vi "SW_Add_or_Modify_Reward_Condition_2.vi"(3 "Array of conditions out":T12, 6 "IO parameters cluster":T1, 7 "Add or Modify?":enum16{"Add", "Modify"}(ring), 8 "error in (no error)":T15, 9 "Main Tree Control in":refnum<vi>, 10 "Calibration parameters":T13={"Timing calibration sw/hw"=1.0, "True FPS"=80.0, "True frame time, s"=0.0125, "Disp. calibration info"=[]} {"True frame time, s" format="%.10g"; "Disp. calibration info"."Speed, µl per ms" format="%.3g"; "True FPS" format="%.10g"; "Timing calibration sw/hw" format="%.10g"}, 11 "Array of conditions in":T12) -> (0 "error out":T15, 1 "Main Tree Control out":refnum<vi>)   [LabVIEW 2018, in "Tracker.lvlib"]
uses:
  Tracker.lvlib
  <vilib>/Utility/miscctls.llb/LVPointTypeDef.ctl
  Controls/CTL_Dispenser_calibration_info.ctl
  Controls/CTL_Calibration_parameters.ctl
  Classes/Reward_Condition/Reward_Condition.lvclass
  Classes/Reward_Condition/Controls/RC_Array_of_Conditions.ctl
  Controls/CTL_Conditions_build_parameters_2.ctl
  Controls/CTL_Condition_type.ctl
  Controls/CTL_Comparison_type.ctl
  Controls/CTL_Validity_check_criteria.ctl
  Controls/CTL_Condition_response_type.ctl
  Controls/CTL_Conditions_Cluster.ctl
  Controls/CTL_IO_params_cluster.ctl
  Controls/CTL_Reponse_port_info.ctl
  Controls/CTL_Response_info.ctl
panel:
  out "Local tree ref":refnum<vi>
  in  "Discard and exit":bool
  in  "Reset Button":bool
  out "Index of selected condition":i32
  out "Has been set":bool
  in  "Specifiers On/Off":T2
  in  "Save and exit":bool
  out "Validity criteria(s)":T4(array[cluster])
  out "Subcondition":T5={"Enabled"=FALSE, "Name"="", "Specifier(s)"=[], "Response"={"Response type"=enum."Air puff", "TTL port"=enum."Port 1", "TTL pulse length, ms"=0.0}, "Has been set"=FALSE} caption="Condition" {"Specifier(s)"."Validity criteria(s)"."Validity value" min=0.0 step=0.1 format="%.2g"; "Specifier(s)"."Value" step=1.0 format="%#.2g"}
  in  "TTL pulse length":dbl caption="No output"
  in  "TTL port":T10
  in  "Response type":T9=enum."Air puff"
  in  "Valid for, units":dbl caption="Has been True for, units" format="%.2g"
  in  "Validity Enabled":bool caption="Enabled"
  in  "SC. Validity Criteria":T3 caption="Validity Criteria"
  in  "Compare against":dbl
  in  "Comparison type":T7
  in  "SubCondition type":T6
  in  "Subcondition #":i32(slide)=5 min=1 max=5 step=1 scale=5.0..1.0
  in  "Specifier(s)":T11(array[cluster])
  in  "C. Name":string caption="Condition Name"
  out "Cond. work index":i32
  in  "C. Enabled":bool caption="Enabled"
  out "Review changes before save":string(tree) caption="Reward and stimulation out"
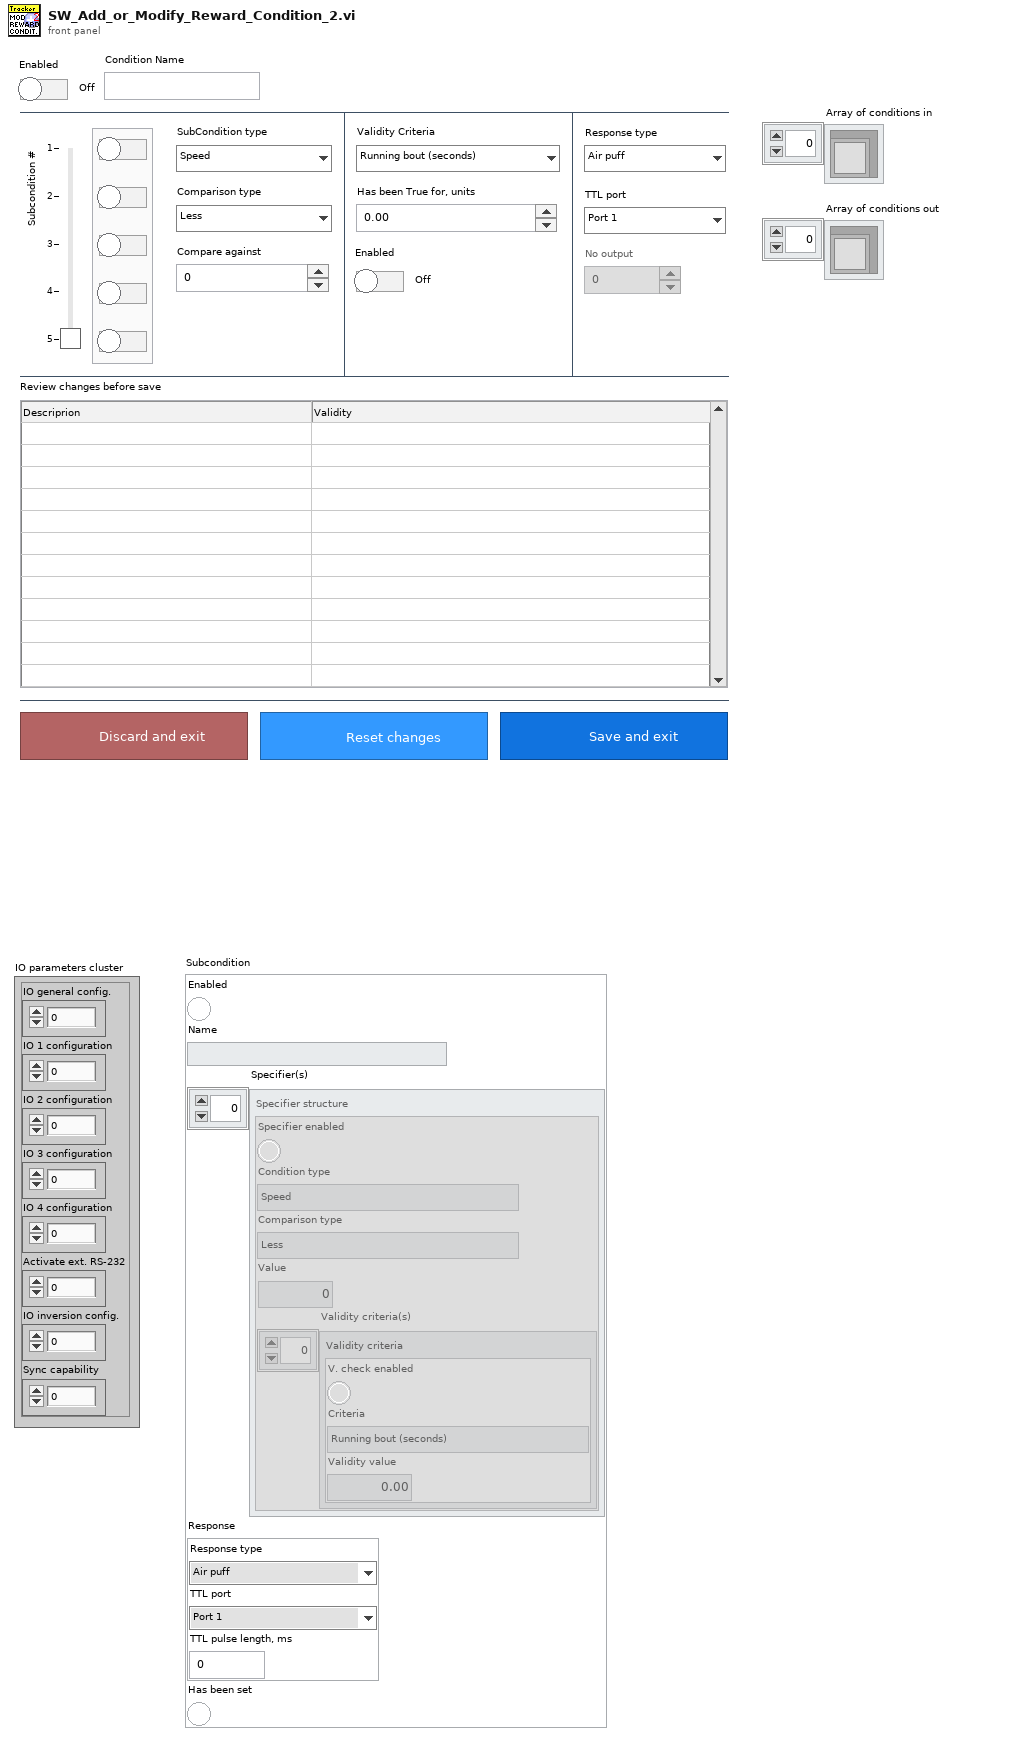
[diagram p1: front panel]
types:
  T1 = typedef "Tracker.lvlib/CTL_IO_params_cluster.ctl" = cluster{"IO general config.":u16, "IO 1 configuration":u16, "IO 2 configuration":u16, "IO 3 configuration":u16, "IO 4 configuration":u16, "Activate ext. RS-232":u16, "IO inversion config.":u16, "Sync capability":u8}
  T2 = cluster{"Specifier on/off":bool, "Specifier on/off 2":bool, "Specifier on/off 3":bool, "Specifier on/off 4":bool, "Specifier on/off 5":bool}
  T3 = typedef "Tracker.lvlib/CTL_Validity_check_criteria.ctl" = enum16{"Running bout (seconds)", "Running bout (meters)"}
  T4 = cluster{"V. check enabled":bool, "Criteria":T3, "Validity value":dbl}[]
  T5 = typedef "Tracker.lvlib/CTL_Conditions_Cluster.ctl" = cluster{"Enabled":bool, "Name":string, "Specifier(s)":cluster{"Specifier enabled":bool, "Condition type":T6, "Comparison type":T7, "Value":dbl, "Validity criteria(s)":cluster{"V. check enabled":bool, "Criteria":T3, "Validity value":dbl}[]}[], "Response":T8, "Has been set":bool}
  T6 = typedef "Tracker.lvlib/CTL_Condition_type.ctl" = enum16{"Speed", "Zone", "Angle to wall"}
  T7 = typedef "Tracker.lvlib/CTL_Comparison_type.ctl" = enum16{"Less", "Less or Equal", "Equal", "Greater or Equal", "Greater", "Not Equal"}
  T8 = typedef "Tracker.lvlib/CTL_Response_info.ctl" = cluster{"Response type":T9, "TTL port":T10, "TTL pulse length, ms":dbl}
  T9 = typedef "Tracker.lvlib/CTL_Condition_response_type.ctl" = enum16{"None", "Air puff", "Liquid reward"}
  T10 = typedef "Tracker.lvlib/CTL_Reponse_port_info.ctl" = enum16{"Port 1", "Port 2", "Port 3", "Port 4"}
  T11 = cluster{"Specifier enabled":bool, "Condition type":T6, "Comparison type":T7, "Value":dbl, "Validity criteria(s)":cluster{"V. check enabled":bool, "Criteria":T3, "Validity value":dbl}[]}[]
  T12 = typedef "Tracker.lvlib/Reward_Condition.lvclass/RC_Array_of_Conditions.ctl" = refnum<class "Reward_Condition.lvclass">[]
  T13 = typedef "Tracker.lvlib/CTL_Calibration_parameters.ctl" = cluster{"Timing calibration sw/hw":dbl, "True FPS":dbl, "True frame time, s":dbl, "Disp. calibration info":T14}
  T14 = typedef "Tracker.lvlib/CTL_Dispenser_calibration_info.ctl" = cluster{"Channel":u8, "Speed, µl per ms":dbl}[]
  T15 = cluster{"Boolean Round":bool, "code":i32, "source":string}
  T16 = typedef "LVPointTypeDef.ctl" = cluster{"Horizontal":i16, "Vertical":i16}
  T17 = typedef "Tracker.lvlib/CTL_Conditions_build_parameters_2.ctl" = cluster{"TreeControl":refnum<vi>, "TTL pulse length ref":refnum<vi>, "Array of conditions":T12, "Condition working index":i32, "Subcondition #":i32, "Calibration parameters":T13}
  T18 = cluster{"[0]":bool, "[1]":bool, "[2]":bool, "[3]":bool, "[4]":bool}
  T19 = cluster{"Specifier enabled":bool, "Condition type":T6, "Comparison type":T7, "Value":dbl, "Validity criteria(s)":cluster{"V. check enabled":bool, "Criteria":T3, "Validity value":dbl}[]}
  T20 = cluster{"V. check enabled":bool, "Criteria":T3, "Validity value":dbl}
  T21 = cluster{"Specifiers On/Off[0]":bool, "Specifiers On/Off[1]":bool, "Specifiers On/Off[2]":bool, "Specifiers On/Off[3]":bool, "Specifiers On/Off[4]":bool}
  T22 = cluster{"Validity Enabled":bool, "SC. Validity Criteria":T3, "Valid for, units":dbl}
  T23 = cluster{"Response type":T9, "TTL port":T10, "TTL pulse length, ms out":dbl}
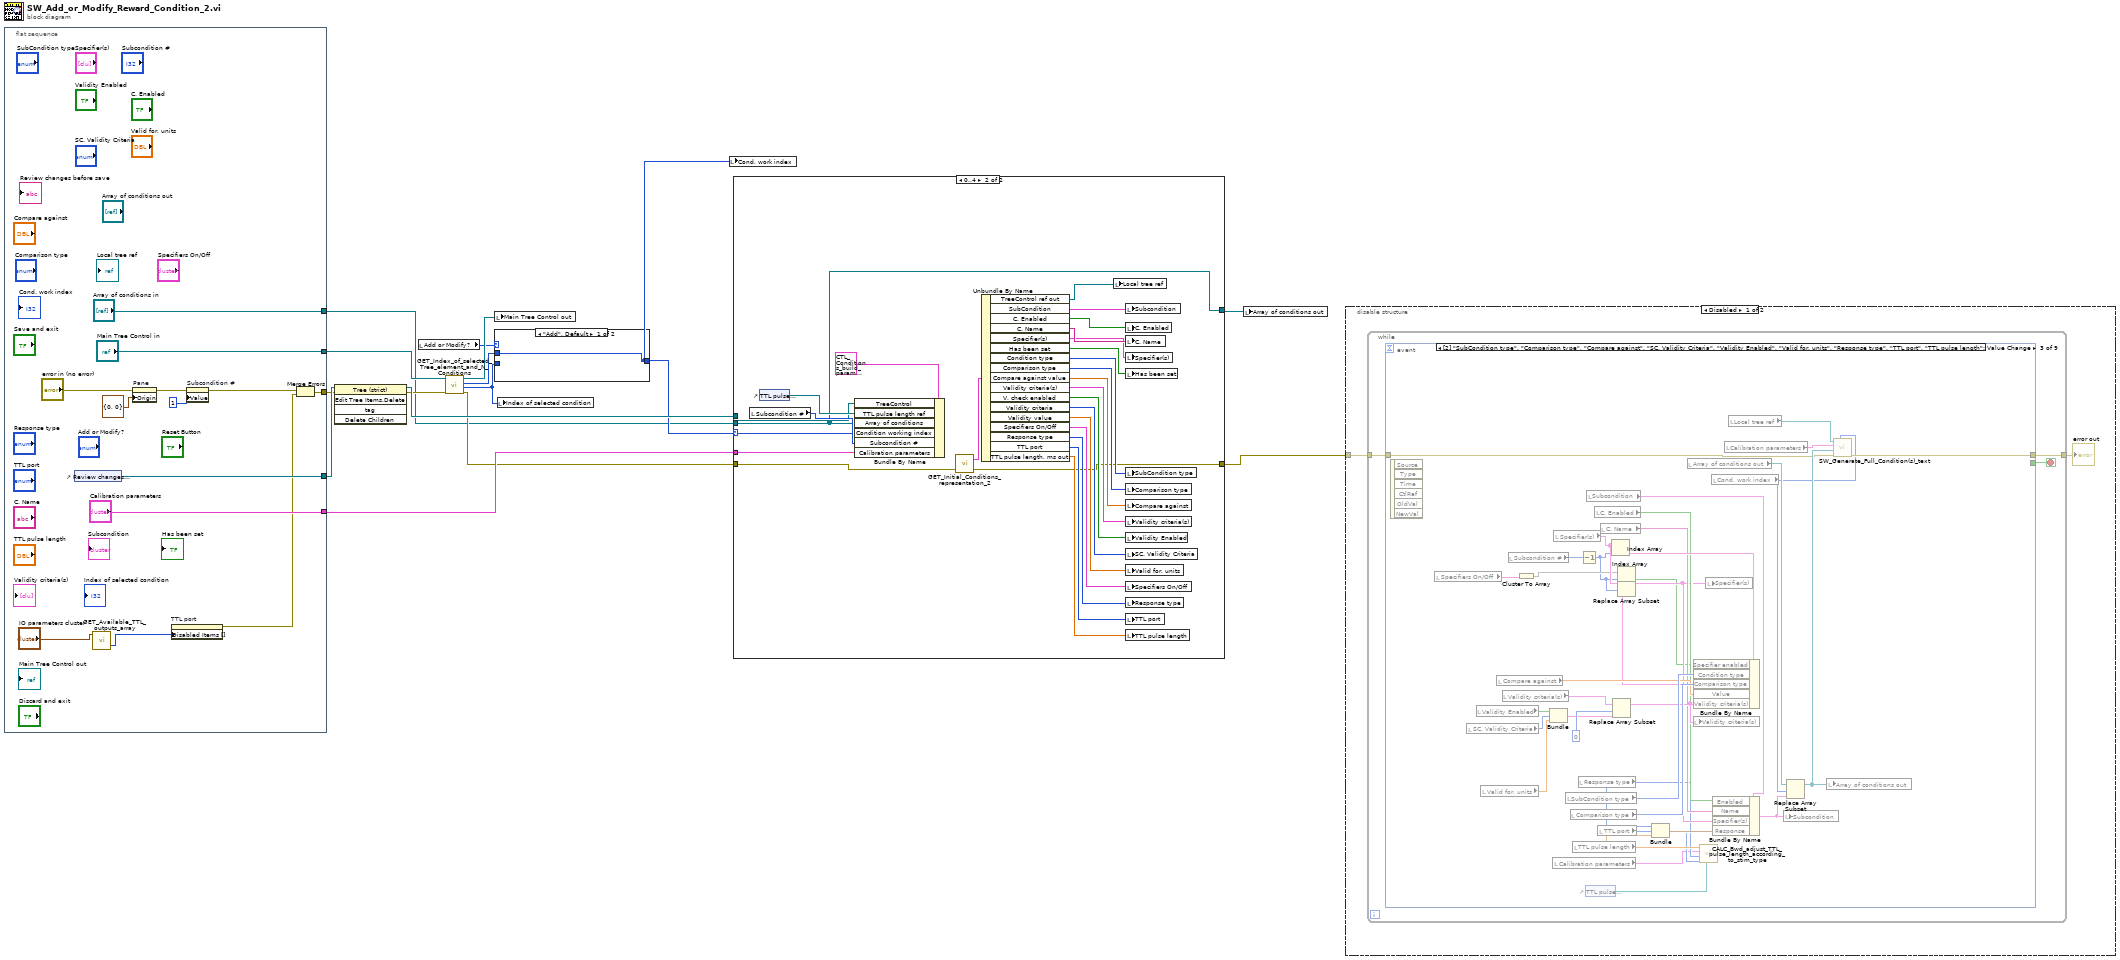
[diagram p0: block diagram]
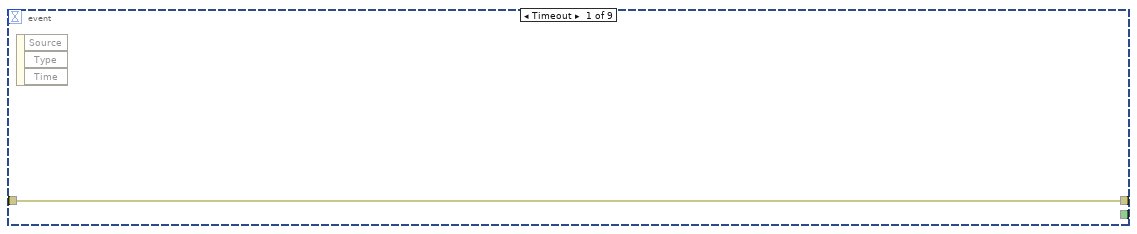
[diagram p2: hidden frame]
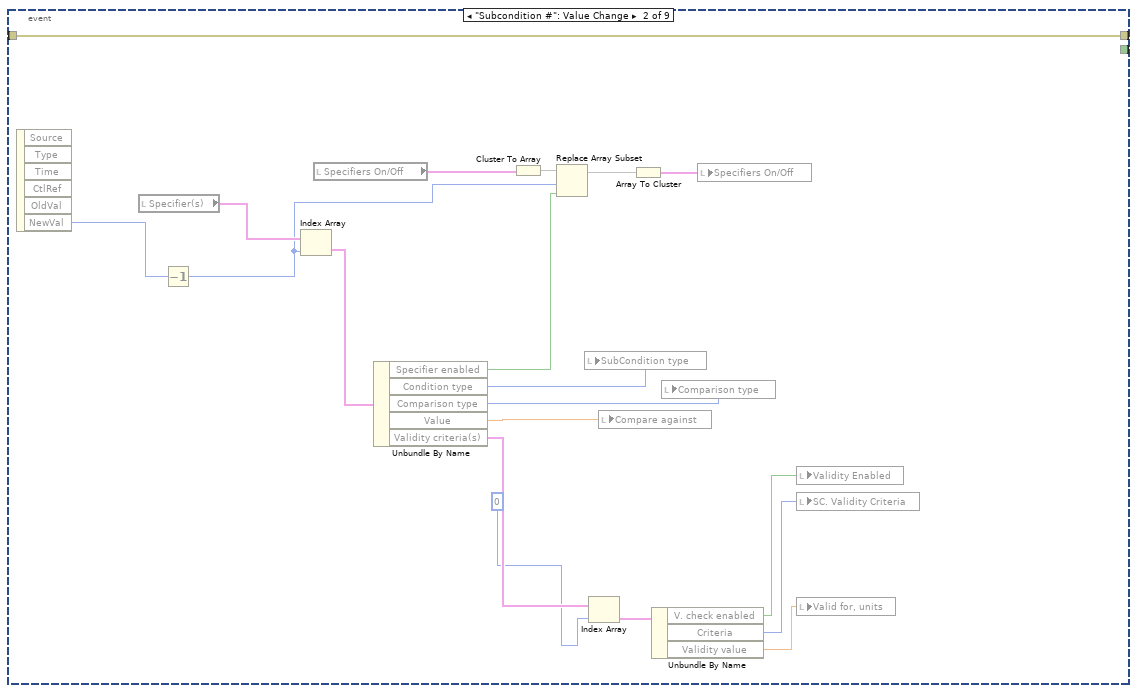
[diagram p3: hidden frame]
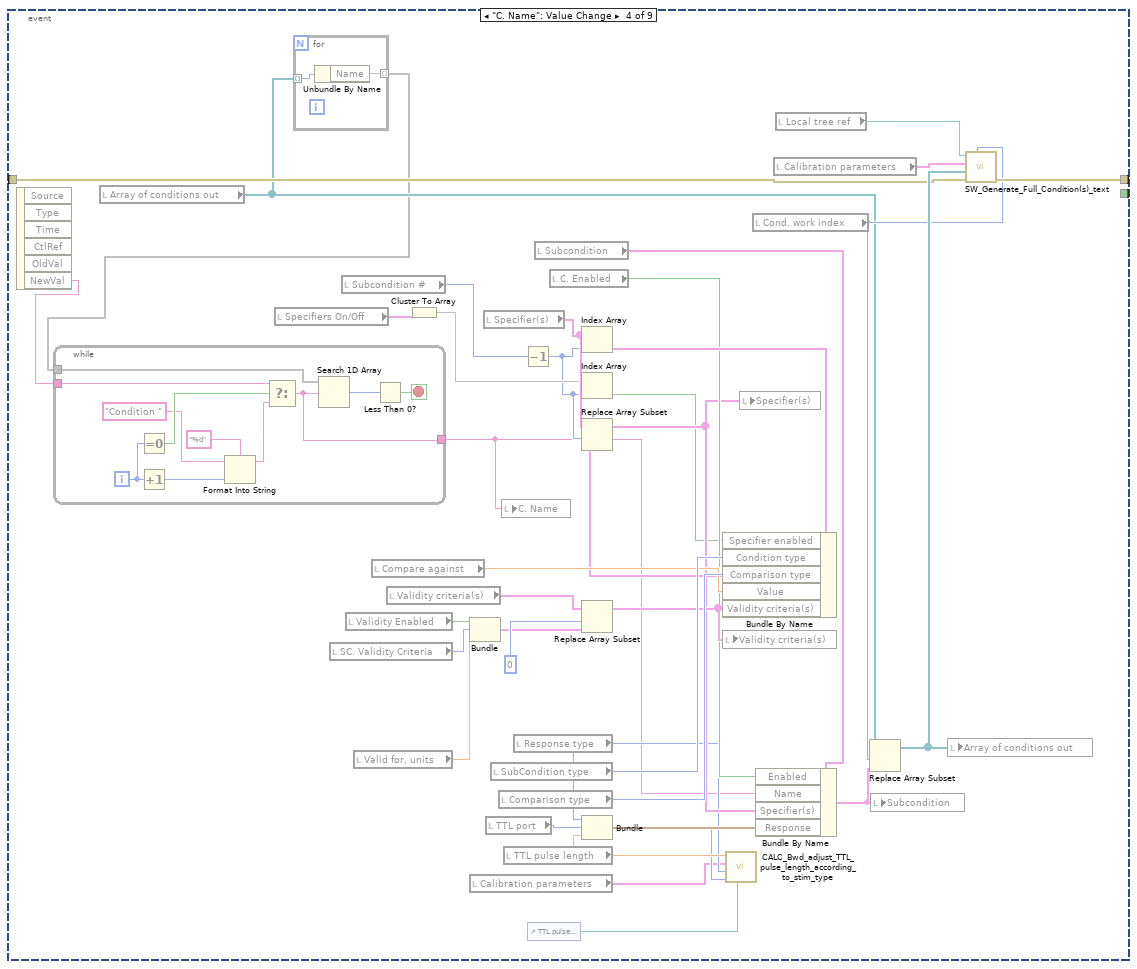
[diagram p4: hidden frame]
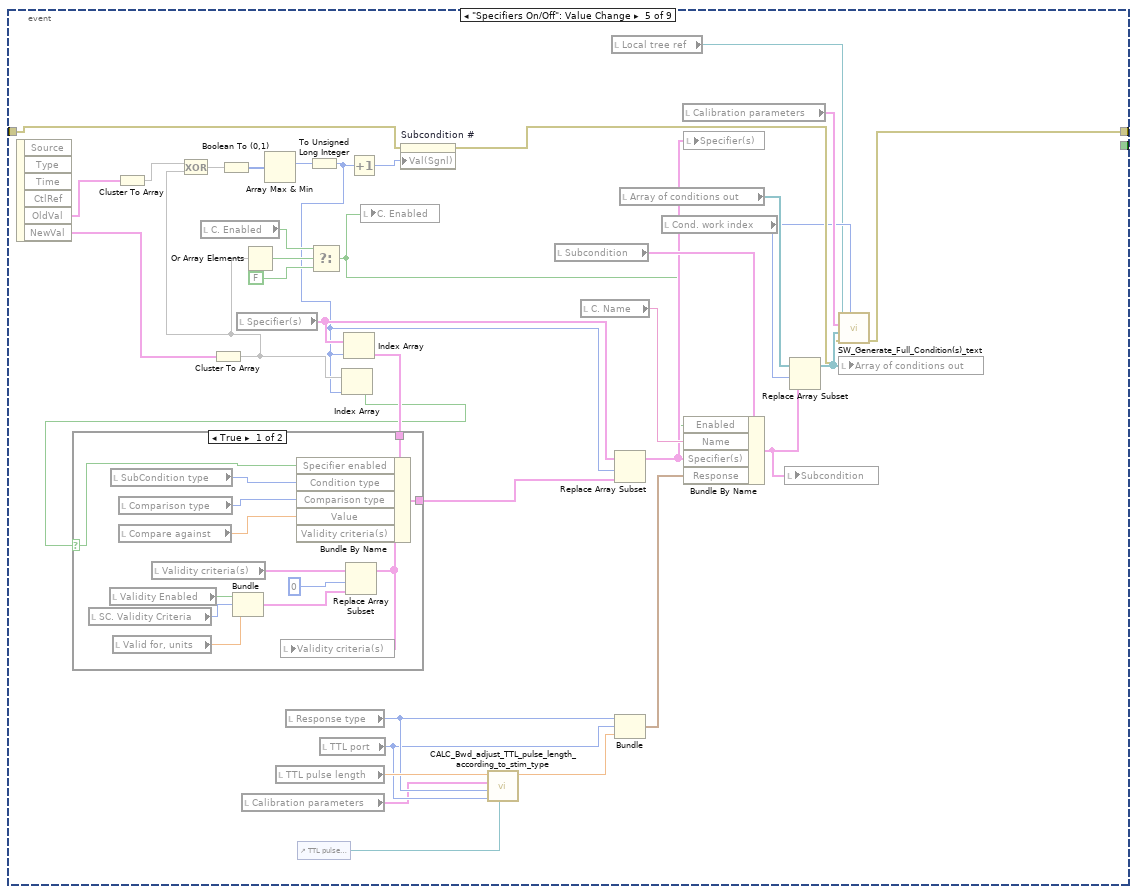
[diagram p5: hidden frame]
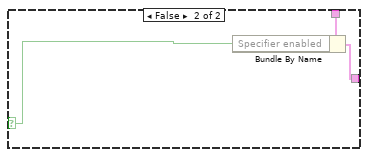
[diagram p6: hidden frame]
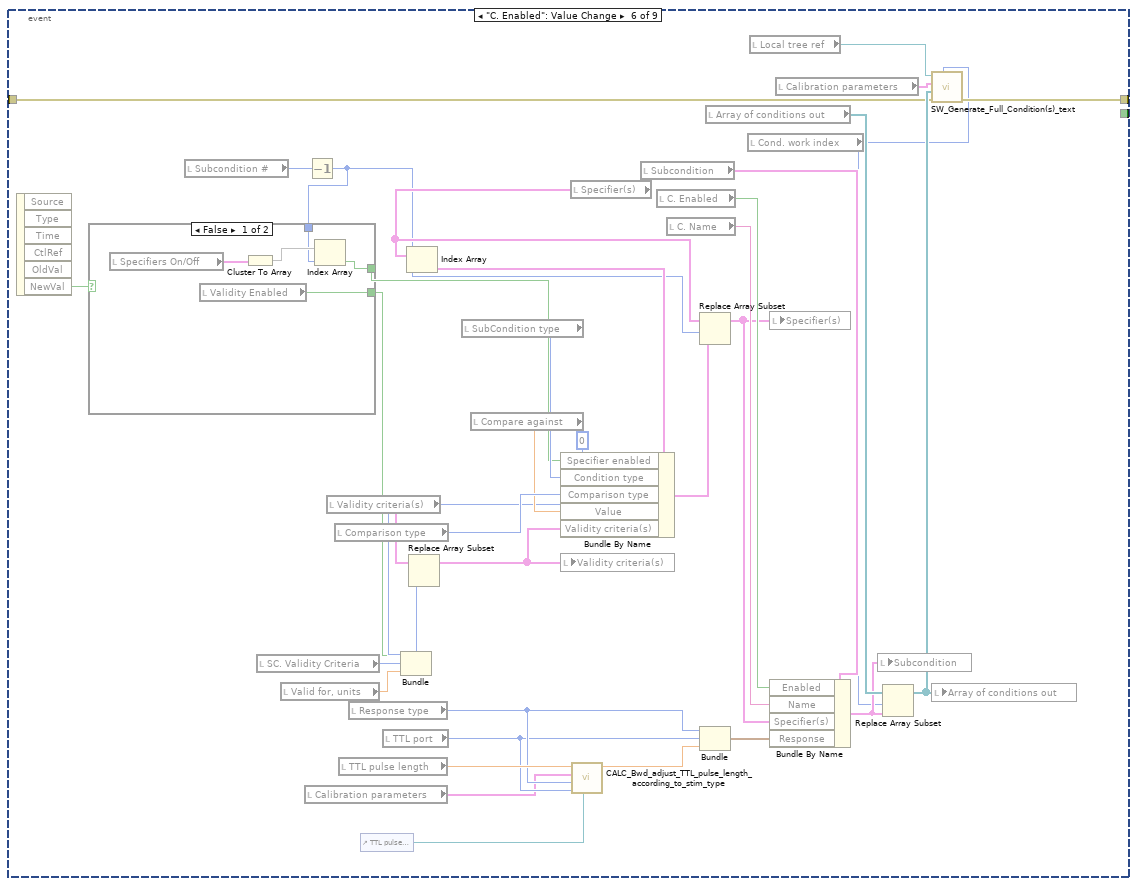
[diagram p7: hidden frame]
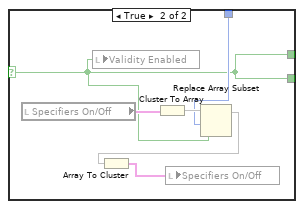
[diagram p8: hidden frame]
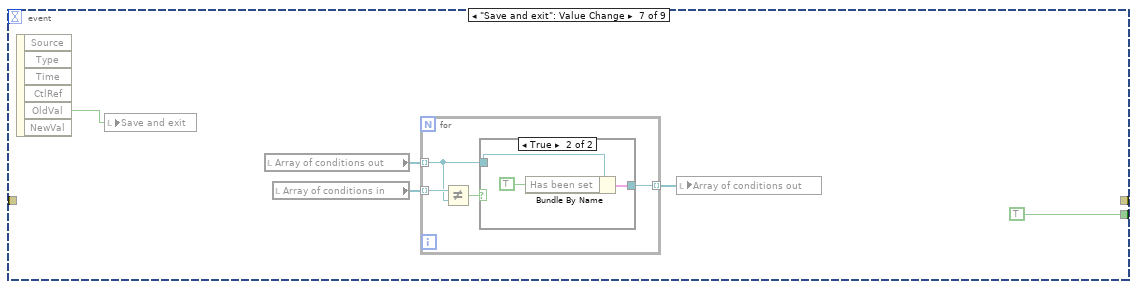
[diagram p9: hidden frame]
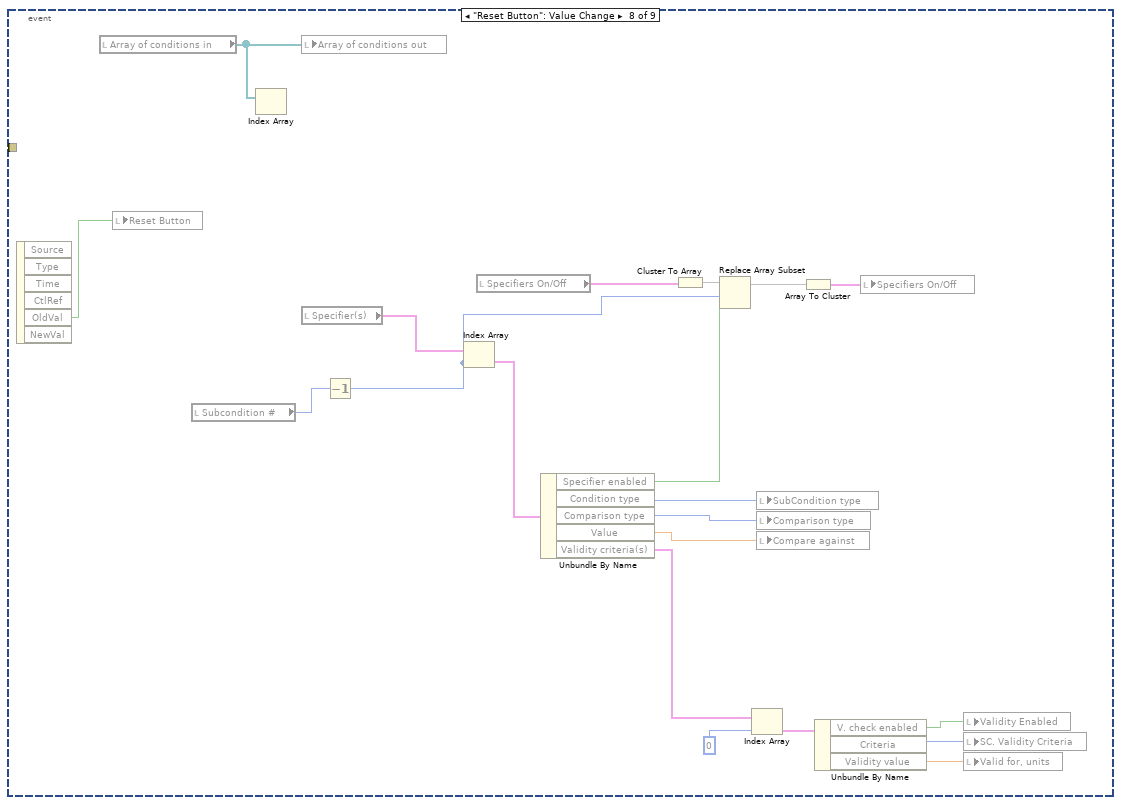
[diagram p11: hidden frame]
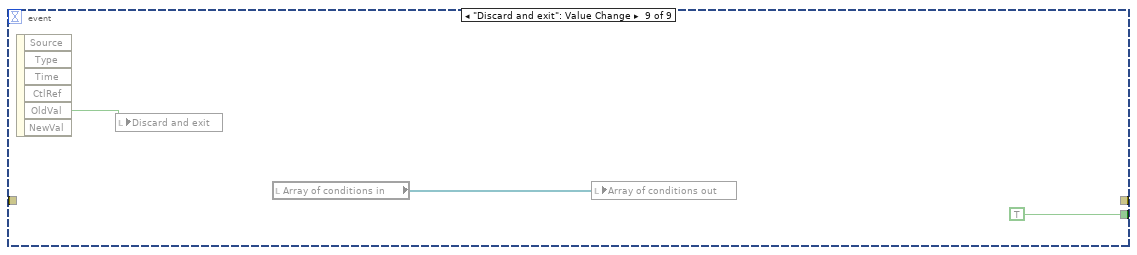
[diagram p12: hidden frame]
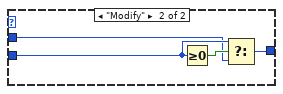
[diagram p15: hidden frame]
diagram:
  n1 = flat-sequence {
    tunnel: [w18] -> w14
    tunnel: [w26] -> w15
    tunnel: ["Main Tree Control in"] -> w4
    tunnel: ["Array of conditions in"] -> w1
    tunnel: ["Calibration parameters"] -> w12
    frame #0 {
      n2 = control-ref of="Review changes before save"() -> (w26:refnum<vi>)
      n3 = call "GET_Available_TTL_outputs_array.vi"("IO parameters cluster"="IO parameters cluster") -> ("Disabled items"=w16:i32[])  [unwired: 2 in, 1 out]
      n4 = property on="Pane" class="Pane"(error in="error in (no error)", "Origin"=T16 {"Horizontal"=0, "Vertical"=0}) -> (error out=w22:errorcluster)  [unwired: 1 in, 1 out]
      n5 = property on="TTL port" class="Enum (strict)"("Disabled Items []"=w16) -> (error out=w17:errorcluster)  [unwired: 2 in, 1 out]
      n6 = property on="Subcondition #" class="Slide (strict)"(error in=w22, "Value"=1 ("Subcondition #")) -> (error out=w21:errorcluster)  [unwired: 1 in, 1 out]
      n7 = Merge Errors(w21, w17) -> (w18:errorcluster)
    }
  }
  n8 = invoke class="Tree (strict)" method="Edit Tree Items.Delete"(reference=w15, error in=w14) -> (reference out=w11:refnum<vi>, error out=w5:errorcluster)  [unwired: 3 in, 3 out]
  n9 = local read "Add or Modify?"() -> (w7:enum16{"Add", "Modify"})
  n10 = call "GET_Index_of_selected_Tree_element_and_N_Conditions.vi"("error in (no error)"=w5, "TreeControl in"=w4) -> ("error out"=w8:errorcluster, "Index of selected element"=w2:i32, "Amount of conditions"=w3:i32, "TreeControl out"=w9:refnum<vi>)  [unwired: 6 in]
  n11 = local write "Main Tree Control out"(w9) -> ()
  n12 = case shown="\"Add\", Default" w7 {
    tunnel: w3 -> [w29 w30]
    tunnel: w2 -> [_ w31]
    tunnel: [w29 w33] -> w6
    frame "Add", Default {
    }
    frame "Modify" {
      n13 = Greater Or Equal To 0?(x=w31) -> (x >= 0?=w32:bool)
      n14 = Select(t=w31, s=w32, f=w30) -> (s? t:f=w33:i32)
    }
  }
  n15 = local write "Index of selected condition"(w2) -> ()
  n16 = local write "Cond. work index"(w6) -> ()
  n17 = case shown="0..4" w6 {
    selector: w6 -> [_ w58]
    tunnel: w1 -> [w35 w56]
    tunnel: [w35 w56] -> w13
    tunnel: w8 -> [w34 w62]
    tunnel: w12 -> [_ w59]
    tunnel: w11 -> [_ w57]
    tunnel: [w34 w38] -> w10
    frame 5.., Default {
    }
    frame 0..4 {
      n18 = local read "Subcondition #"() -> (w60:i32)
      n19 = control-ref of="TTL pulse length"() -> (w61:refnum<vi>)
      n20 = Bundle By Name(cluster=T17 {"TreeControl"=refnum, "TTL pulse length ref"=refnum, "Array of conditions"=[], "Condition working index"=0, "Subcondition #"=0, "Calibration parameters"={"Timing calibration sw/hw"=0.0, "True FPS"=0.0, "True frame time, s"=0.0, "Disp. calibration info"=[]}} ("Input parameters cluster"), "TreeControl"=w57, "TTL pulse length ref"=w61, "Array of conditions"=w56, "Condition working index"=w58, "Subcondition #"=w60, "Calibration parameters"=w59) -> ()  [unwired: 1 out]
      n21 = call "GET_Initial_Conditions_representation_2.vi"("error in (no error)"=w62) -> ("error out"=w38:errorcluster, "Output parameters cluster"=w55:T17)  [unwired: 1 in]
      n22 = Unbundle By Name(w55) -> ("TreeControl ref out"=w37:refnum<vi>, "SubCondition"=w50:T5, "C. Enabled"=w49:bool, "C. Name"=w48:string, "Specifier(s)"=w47:T11, "Has been set"=w39:bool, "Condition type"=w46:T6, "Comparison type"=w40:T7, "Compare against value"=w42:dbl, "Validity criteria(s)"=w41:T4, "V. check enabled"=w44:bool, "Validity criteria"=w45:T3, "Validity value"=w43:dbl, "Specifiers On/Off"=w51:T18, "Response type"=w54:T9, "TTL port"=w52:T10, "TTL pulse length, ms out"=w53:dbl)
      n23 = local write "Local tree ref"(w37) -> ()
      n24 = local write "Subcondition"(w50) -> ()
      n25 = local write "C. Enabled"(w49) -> ()
      n26 = local write "C. Name"(w48) -> ()
      n27 = local write "Specifier(s)"(w47) -> ()
      n28 = local write "Has been set"(w39) -> ()
      n29 = local write "SubCondition type"(w46) -> ()
      n30 = local write "Comparison type"(w40) -> ()
      n31 = local write "Compare against"(w42) -> ()
      n32 = local write "Validity criteria(s)"(w41) -> ()
      n33 = local write "Validity Enabled"(w44) -> ()
      n34 = local write "SC. Validity Criteria"(w45) -> ()
      n35 = local write "Valid for, units"(w43) -> ()
      n36 = local write "Specifiers On/Off"(w51) -> ()
      n37 = local write "Response type"(w54) -> ()
      n38 = local write "TTL port"(w52) -> ()
      n39 = local write "TTL pulse length"(w53) -> ()
    }
  }
  n40 = local write "Array of conditions out"(w13) -> ()
  n41 = disable-structure shown="Disabled" {
    disable-tunnel: w10 -> [w63 _]
    frame Disabled {
      n42 = while {
        tunnel: w63 -> [w67]
        tunnel: [w66] -> w64
        stop <- w65 stop-if-true
        n43 = event shown="[2] \"SubCondition type\", \"Comparison type\", \"Compare against\", \"SC. Validity Criteria\", \"Validity Enabled\", \"Valid for, units\", \"Response type\", \"TTL port\", \"TTL pulse length\": Value Change" {
          selector: _ -> [_ _ _ _ _ _ _ _ _]
          dyn-events: _ -> [_ _ _ _ _ _ _ _ _]
          timeout: _ -> [_ _ _ _ _ _ _ _ _]
          tunnel: w67 -> [w68 w86 w102 w143 w183 w243 _ _ _]
          tunnel: [w68 w86 w101 w142 w201 w242 _ _ _] -> w66
          tunnel: [_ _ _ _ _ _ TRUE _ TRUE] -> w65
          event Timeout {
            n44 = event-data() -> ()  [unwired: 1 in, 3 out]
          }
          event "Subcondition #": Value Change {
            n45 = event-data() -> ("NewVal"=w87:i32)  [unwired: 1 in, 5 out]
            n46 = local read "Specifier(s)"() -> (w85:T11)
            n47 = Decrement(x=w87) -> (x-1=w69:i32)
            n48 = Index Array(array=w85, index=w69) -> (element=w84:T19)
            n49 = local read "Specifiers On/Off"() -> (w74:T2)
            n50 = Unbundle By Name(w84) -> ("Specifier enabled"=w70:bool, "Condition type"=w83:T6, "Comparison type"=w82:T7, "Value"=w81:dbl, "Validity criteria(s)"=w80:T4)
            n51 = Cluster To Array(cluster=w74) -> (array=w73:bool[])
            n52 = Replace Array Subset(array=w73, new element=w70, index=w69) -> (w72:bool[])
            n53 = local write "SubCondition type"(w83) -> ()
            n54 = Index Array(array=w80, index=0) -> (element=w78:T20)
            n55 = local write "Compare against"(w81) -> ()
            n56 = Array To Cluster(array=w72) -> (cluster=w71:T21)
            n57 = Unbundle By Name(w78) -> ("V. check enabled"=w76:bool, "Criteria"=w77:T3, "Validity value"=w75:dbl)
            n58 = local write "Comparison type"(w82) -> ()
            n59 = local write "Specifiers On/Off"(w71) -> ()
            n60 = local write "Validity Enabled"(w76) -> ()
            n61 = local write "SC. Validity Criteria"(w77) -> ()
            n62 = local write "Valid for, units"(w75) -> ()
          }
          event "Compare against", "Validity Enabled", "Valid for, units", "TTL pulse length": Value Change {
            n63 = event-data() -> ()  [unwired: 1 in, 6 out]
            n64 = local read "Specifiers On/Off"() -> (w94:T2)
            n65 = local read "SC. Validity Criteria"() -> (w117:T3)
            n66 = local read "Validity Enabled"() -> (w118:bool)
            n67 = local read "Valid for, units"() -> (w116:dbl)
            n68 = local read "Compare against"() -> (w121:dbl)
            n69 = local read "Validity criteria(s)"() -> (w120:T4)
            n70 = local read "Subcondition #"() -> (w89:i32)
            n71 = Cluster To Array(cluster=w94) -> (array=w93:bool[])
            n72 = Bundle("Validity Enabled"=w118, "SC. Validity Criteria"=w117, "Valid for, units"=w116) -> (w115:T22)  [unwired: 1 in]
            n73 = local read "Calibration parameters"() -> (w96:T13)
            n74 = local read "Specifier(s)"() -> (w113:T11)
            n75 = local read "SubCondition type"() -> (w123:T6)
            n76 = local read "Comparison type"() -> (w122:T7)
            n77 = local read "TTL pulse length"() -> (w100:dbl)
            n78 = local read "Response type"() -> (w99:T9)
            n79 = Decrement(x=w89) -> (x-1=w91:i32)
            n80 = control-ref of="TTL pulse length"() -> (w95:refnum<vi>)
            n81 = local read "Subcondition"() -> (w108:T5)
            n82 = local read "C. Enabled"() -> (w109:bool)
            n83 = local read "TTL port"() -> (w98:T10)
            n84 = local read "C. Name"() -> (w110:string)
            n85 = Index Array(array=w113, index=w91) -> (element=w124:T19)
            n86 = Replace Array Subset(array=w120, new element=w115, index=0) -> (w114:T4)
            n87 = Index Array(array=w93, index=w91) -> (element=w92:bool)
            n88 = local read "Array of conditions out"() -> (w106:T12)
            n89 = Bundle By Name(cluster=w124, "Specifier enabled"=w92, "Condition type"=w123, "Comparison type"=w122, "Value"=w121, "Validity criteria(s)"=w114) -> (w112:T19)
            n90 = Replace Array Subset(array=w113, new element=w112, index=w91) -> (w107:T11)
            n91 = local write "Validity criteria(s)"(w114) -> ()
            n92 = call "CALC_Bwd_adjust_TTL_pulse_length_according_to_stim_type.vi"("TTL pulse length ref in"=w95, "TTL port"=w98, "Response type"=w99, "Calibration parameters"=w96, "TTL pulse length, units, in"=w100) -> ("TTL pulse length, ms out"=w97:dbl)  [unwired: 6 in]
            n93 = Bundle("Response type"=w99, "TTL port"=w98, "TTL pulse length, ms out"=w97) -> (w111:T23)  [unwired: 1 in]
            n94 = local write "Specifier(s)"(w107) -> ()
            n95 = local read "Cond. work index"() -> (w90:i32)
            n96 = Bundle By Name(cluster=w108, "Enabled"=w109, "Name"=w110, "Specifier(s)"=w107, "Response"=w111) -> (w105:T5)
            n97 = local read "Calibration parameters"() -> (w103:T13)
            n98 = local read "Local tree ref"() -> (w88:refnum<vi>)
            n99 = local write "Subcondition"(w105) -> ()
            n100 = Replace Array Subset(array=w106, new element=w105, index=w90) -> (w104:T12)
            n101 = local write "Array of conditions out"(w104) -> ()
            n102 = call "SW_Generate_Full_Condition(s)_text.vi"("Array index to show"=w90, "error in (no error)"=w102, "Array of conditions in"=w104, "Calibration parameters"=w103, "TreeControl ref in"=w88) -> ("error out"=w101:errorcluster)  [unwired: 5 in, 1 out]
          }
          event "C. Name": Value Change {
            n103 = event-data() -> ("NewVal"=w129:string)  [unwired: 1 in, 5 out]
            n104 = local read "Array of conditions out"() -> (w128:T12)
            n105 = local read "Specifiers On/Off"() -> (w135:T2)
            n106 = for {
              tunnel: w128 -> [w165] mode=indexing
              tunnel: [w164] -> w127 mode=indexing
              n107 = Unbundle By Name(w165) -> ("Name"=w164)
            }
            n108 = while {
              tunnel: w127 -> [w175]
              tunnel: [w166] -> w126
              tunnel: w129 -> [w167]
              i -> [w169]
              stop <- w174 stop-if-true
              n109 = Equal To 0?(x=w169) -> (x = 0?=w173:bool)
              n110 = Increment(x=w169) -> (x+1=w172:i32)
              n111 = Format Into String(format string="%d", initial string="Condition ", w172) -> (resulting string=w168:string)  [unwired: 1 in, 1 out]
              n112 = Select(t=w167, s=w173, f=w168) -> (s? t:f=w166:string)
              n113 = Search 1D Array(1D array=w175, element=w166) -> (index of element=w176:i32)  [unwired: 1 in]
              n114 = Less Than 0?(x=w176) -> (x < 0?=w174:bool)
            }
            n115 = local read "SC. Validity Criteria"() -> (w156:T3)
            n116 = local read "Subcondition #"() -> (w130:i32)
            n117 = local read "Validity Enabled"() -> (w157:bool)
            n118 = local read "Valid for, units"() -> (w155:dbl)
            n119 = local read "Compare against"() -> (w160:dbl)
            n120 = local read "Validity criteria(s)"() -> (w159:T4)
            n121 = Cluster To Array(cluster=w135) -> (array=w134:bool[])
            n122 = Bundle("Validity Enabled"=w157, "SC. Validity Criteria"=w156, "Valid for, units"=w155) -> (w154:T22)  [unwired: 1 in]
            n123 = local read "Calibration parameters"() -> (w137:T13)
            n124 = local read "Specifier(s)"() -> (w152:T11)
            n125 = local read "TTL port"() -> (w139:T10)
            n126 = local read "SubCondition type"() -> (w162:T6)
            n127 = local read "Comparison type"() -> (w161:T7)
            n128 = local write "C. Name"(w126) -> ()
            n129 = local read "TTL pulse length"() -> (w141:dbl)
            n130 = local read "Response type"() -> (w140:T9)
            n131 = Decrement(x=w130) -> (x-1=w132:i32)
            n132 = control-ref of="TTL pulse length"() -> (w136:refnum<vi>)
            n133 = local read "Subcondition"() -> (w148:T5)
            n134 = local read "C. Enabled"() -> (w149:bool)
            n135 = Index Array(array=w152, index=w132) -> (element=w163:T19)
            n136 = Index Array(array=w134, index=w132) -> (element=w133:bool)
            n137 = Replace Array Subset(array=w159, new element=w154, index=0) -> (w153:T4)
            n138 = Bundle By Name(cluster=w163, "Specifier enabled"=w133, "Condition type"=w162, "Comparison type"=w161, "Value"=w160, "Validity criteria(s)"=w153) -> (w151:T19)
            n139 = Replace Array Subset(array=w152, new element=w151, index=w132) -> (w147:T11)
            n140 = local write "Validity criteria(s)"(w153) -> ()
            n141 = call "CALC_Bwd_adjust_TTL_pulse_length_according_to_stim_type.vi"("TTL pulse length ref in"=w136, "TTL port"=w139, "Response type"=w140, "Calibration parameters"=w137, "TTL pulse length, units, in"=w141) -> ("TTL pulse length, ms out"=w138:dbl)  [unwired: 6 in]
            n142 = Bundle("Response type"=w140, "TTL port"=w139, "TTL pulse length, ms out"=w138) -> (w150:T23)  [unwired: 1 in]
            n143 = local write "Specifier(s)"(w147) -> ()
            n144 = local read "Cond. work index"() -> (w131:i32)
            n145 = Bundle By Name(cluster=w148, "Enabled"=w149, "Name"=w126, "Specifier(s)"=w147, "Response"=w150) -> (w146:T5)
            n146 = local read "Calibration parameters"() -> (w144:T13)
            n147 = local read "Local tree ref"() -> (w125:refnum<vi>)
            n148 = Replace Array Subset(array=w128, new element=w146, index=w131) -> (w145:T12)
            n149 = local write "Subcondition"(w146) -> ()
            n150 = local write "Array of conditions out"(w145) -> ()
            n151 = call "SW_Generate_Full_Condition(s)_text.vi"("Array index to show"=w131, "error in (no error)"=w143, "Array of conditions in"=w145, "Calibration parameters"=w144, "TreeControl ref in"=w125) -> ("error out"=w142:errorcluster)  [unwired: 5 in, 1 out]
          }
          event "Specifiers On/Off": Value Change {
            n152 = event-data() -> ("OldVal"=w189:T2, "NewVal"=w190:T2)  [unwired: 1 in, 4 out]
            n153 = Cluster To Array(cluster=w189) -> (array=w188:bool[])
            n154 = local read "C. Enabled"() -> (w192:bool)
            n155 = Cluster To Array(cluster=w190) -> (array=w187:bool[])
            n156 = Exclusive Or(1:w187, 2:w188) -> (0:w186:bool[])
            n157 = Boolean To (0,1)(Boolean=w186) -> (0, 1=w185:i16[])
            n158 = local read "Specifier(s)"() -> (w211:T11)
            n159 = local read "Calibration parameters"() -> (w196:T13)
            n160 = Or Array Elements(Boolean array=w187) -> (logical OR=w194:bool)
            n161 = Array Max & Min(array=w185) -> (max index (indices)=w184:i32)  [unwired: 3 out]
            n162 = local read "TTL pulse length"() -> (w200:dbl)
            n163 = local read "Response type"() -> (w199:T9)
            n164 = control-ref of="TTL pulse length"() -> (w195:refnum<vi>)
            n165 = To Unsigned Long Integer(number=w184) -> (unsigned 32bit integer=w180:u32)
            n166 = Select(t=w192, s=w194, f=FALSE) -> (s? t:f=w191:bool)
            n167 = local read "TTL port"() -> (w198:T10)
            n168 = Index Array(array=w187, index=w180) -> (element=w181:bool)
            n169 = Index Array(array=w211, index=w180) -> (element=w212:T19)
            n170 = case shown="True" w181 {
              selector: w181 -> [w213 w226]
              tunnel: w212 -> [w225 w228]
              tunnel: [w214 w227] -> w210
              frame True {
                n171 = local read "SC. Validity Criteria"() -> (w218:T3)
                n172 = local read "Validity Enabled"() -> (w219:bool)
                n173 = local read "SubCondition type"() -> (w224:T6)
                n174 = local read "Valid for, units"() -> (w217:dbl)
                n175 = local read "Comparison type"() -> (w223:T7)
                n176 = local read "Compare against"() -> (w222:dbl)
                n177 = local read "Validity criteria(s)"() -> (w221:T4)
                n178 = Bundle("Validity Enabled"=w219, "SC. Validity Criteria"=w218, "Valid for, units"=w217) -> (w216:T22)  [unwired: 1 in]
                n179 = Replace Array Subset(array=w221, new element=w216, index=0) -> (w215:T4)
                n180 = local write "Validity criteria(s)"(w215) -> ()
                n181 = Bundle By Name(cluster=w225, "Specifier enabled"=w213, "Condition type"=w224, "Comparison type"=w223, "Value"=w222, "Validity criteria(s)"=w215) -> (w214:T19)
              }
              frame False {
                n182 = Bundle By Name(cluster=w228, "Specifier enabled"=w226) -> (w227:T19)
              }
            }
            n183 = Increment(x=w180) -> (x+1=w179:u32)
            n184 = local write "C. Enabled"(w191) -> ()
            n185 = property on="Subcondition #" class="Slide (strict)"(error in=w183, "Val(Sgnl)"=w179) -> (error out=w182:errorcluster)  [unwired: 1 in, 1 out]
            n186 = call "CALC_Bwd_adjust_TTL_pulse_length_according_to_stim_type.vi"("TTL pulse length ref in"=w195, "TTL port"=w198, "Response type"=w199, "Calibration parameters"=w196, "TTL pulse length, units, in"=w200) -> ("TTL pulse length, ms out"=w197:dbl)  [unwired: 6 in]
            n187 = local read "Subcondition"() -> (w207:T5)
            n188 = local read "C. Name"() -> (w208:string)
            n189 = local read "Local tree ref"() -> (w177:refnum<vi>)
            n190 = Replace Array Subset(array=w211, new element=w210, index=w180) -> (w206:T11)
            n191 = Bundle("Response type"=w199, "TTL port"=w198, "TTL pulse length, ms out"=w197) -> (w209:T23)  [unwired: 1 in]
            n192 = local read "Array of conditions out"() -> (w205:T12)
            n193 = local read "Cond. work index"() -> (w178:i32)
            n194 = local read "Calibration parameters"() -> (w202:T13)
            n195 = local write "Specifier(s)"(w206) -> ()
            n196 = Bundle By Name(cluster=w207, "Enabled"=w191, "Name"=w208, "Specifier(s)"=w206, "Response"=w209) -> (w204:T5)
            n197 = local write "Subcondition"(w204) -> ()
            n198 = Replace Array Subset(array=w205, new element=w204, index=w178) -> (w203:T12)
            n199 = call "SW_Generate_Full_Condition(s)_text.vi"("Array index to show"=w178, "error in (no error)"=w182, "Array of conditions in"=w203, "Calibration parameters"=w202, "TreeControl ref in"=w177) -> ("error out"=w201:errorcluster)  [unwired: 5 in, 1 out]
            n200 = local write "Array of conditions out"(w203) -> ()
          }
          event "C. Enabled": Value Change {
            n201 = event-data() -> ("NewVal"=w235:bool)  [unwired: 1 in, 5 out]
            n202 = local read "Subcondition #"() -> (w231:i32)
            n203 = local read "SC. Validity Criteria"() -> (w258:T3)
            n204 = local read "Valid for, units"() -> (w257:dbl)
            n205 = local read "Calibration parameters"() -> (w237:T13)
            n206 = Decrement(x=w231) -> (x-1=w232:i32)
            n207 = case shown="False" w235 {
              selector: w235 -> [_ w272]
              tunnel: [w266 w272] -> w234
              tunnel: [w269 w272] -> w233
              tunnel: w232 -> [w265 w273]
              frame False {
                n208 = local read "Specifiers On/Off"() -> (w268:T2)
                n209 = local read "Validity Enabled"() -> (w269:bool)
                n210 = Cluster To Array(cluster=w268) -> (array=w267:bool[])
                n211 = Index Array(array=w267, index=w265) -> (element=w266:bool)
              }
              frame True {
                n212 = local read "Specifiers On/Off"() -> (w275:T2)
                n213 = local write "Validity Enabled"(w272) -> ()
                n214 = Cluster To Array(cluster=w275) -> (array=w274:bool[])
                n215 = Replace Array Subset(array=w274, new element=w272, index=w273) -> (w271:bool[])
                n216 = Array To Cluster(array=w271) -> (cluster=w270:T21)
                n217 = local write "Specifiers On/Off"(w270) -> ()
              }
            }
            n218 = local read "Validity criteria(s)"() -> (w260:T4)
            n219 = local read "Comparison type"() -> (w262:T7)
            n220 = local read "TTL pulse length"() -> (w241:dbl)
            n221 = local read "Response type"() -> (w240:T9)
            n222 = control-ref of="TTL pulse length"() -> (w236:refnum<vi>)
            n223 = local read "TTL port"() -> (w239:T10)
            n224 = Bundle("Validity Enabled"=w233, "SC. Validity Criteria"=w258, "Valid for, units"=w257) -> (w256:T22)  [unwired: 1 in]
            n225 = Replace Array Subset(array=w260, new element=w256, index=0) -> (w255:T4)
            n226 = local read "SubCondition type"() -> (w263:T6)
            n227 = local read "Compare against"() -> (w261:dbl)
            n228 = local write "Validity criteria(s)"(w255) -> ()
            n229 = local read "Specifier(s)"() -> (w254:T11)
            n230 = Index Array(array=w254, index=w232) -> (element=w264:T19)
            n231 = Bundle By Name(cluster=w264, "Specifier enabled"=w234, "Condition type"=w263, "Comparison type"=w262, "Value"=w261, "Validity criteria(s)"=w255) -> (w253:T19)
            n232 = call "CALC_Bwd_adjust_TTL_pulse_length_according_to_stim_type.vi"("TTL pulse length ref in"=w236, "TTL port"=w239, "Response type"=w240, "Calibration parameters"=w237, "TTL pulse length, units, in"=w241) -> ("TTL pulse length, ms out"=w238:dbl)  [unwired: 6 in]
            n233 = local read "Subcondition"() -> (w249:T5)
            n234 = local read "C. Enabled"() -> (w250:bool)
            n235 = local read "C. Name"() -> (w251:string)
            n236 = Replace Array Subset(array=w254, new element=w253, index=w232) -> (w248:T11)
            n237 = Bundle("Response type"=w240, "TTL port"=w239, "TTL pulse length, ms out"=w238) -> (w252:T23)  [unwired: 1 in]
            n238 = local read "Array of conditions out"() -> (w247:T12)
            n239 = local read "Cond. work index"() -> (w230:i32)
            n240 = local read "Local tree ref"() -> (w229:refnum<vi>)
            n241 = local write "Specifier(s)"(w248) -> ()
            n242 = Bundle By Name(cluster=w249, "Enabled"=w250, "Name"=w251, "Specifier(s)"=w248, "Response"=w252) -> (w246:T5)
            n243 = local read "Calibration parameters"() -> (w244:T13)
            n244 = local write "Subcondition"(w246) -> ()
            n245 = Replace Array Subset(array=w247, new element=w246, index=w230) -> (w245:T12)
            n246 = call "SW_Generate_Full_Condition(s)_text.vi"("Array index to show"=w230, "error in (no error)"=w243, "Array of conditions in"=w245, "Calibration parameters"=w244, "TreeControl ref in"=w229) -> ("error out"=w242:errorcluster)  [unwired: 5 in, 1 out]
            n247 = local write "Array of conditions out"(w245) -> ()
          }
          event "Save and exit": Value Change {
            n248 = event-data() -> ("OldVal"=w280:bool)  [unwired: 1 in, 5 out]
            n249 = local write "Save and exit"(w280) -> ()
            n250 = local read "Array of conditions out"() -> (w277:T12)
            n251 = local read "Array of conditions in"() -> (w278:T12)
            n252 = for {
              tunnel: w278 -> [w284] mode=indexing
              tunnel: w277 -> [w283] mode=indexing
              tunnel: [w282] -> w276 mode=indexing
              n253 = Not Equal?(x=w284, y=w283) -> (x != y?=w281:bool)
              n254 = case shown="True" w281 {
                tunnel: w283 -> [w285 w288]
                tunnel: [w285 w286] -> w282
                frame False {
                }
                frame True {
                  n255 = Bundle By Name(cluster=w288, "Has been set"=TRUE) -> (w286:cluster{})
                }
              }
            }
            n256 = local write "Array of conditions out"(w276) -> ()
          }
          event "Reset Button": Value Change {
            n257 = event-data() -> ("OldVal"=w292:bool)  [unwired: 1 in, 5 out]
            n258 = local read "Array of conditions in"() -> (w289:T12)
            n259 = local write "Reset Button"(w292) -> ()
            n260 = local read "Subcondition #"() -> (w291:i32)
            n261 = Index Array(array=w289) -> ()  [unwired: 1 in, 1 out]
            n262 = local write "Array of conditions out"(w289) -> ()
            n263 = local read "Specifier(s)"() -> (w308:T11)
            n264 = Decrement(x=w291) -> (x-1=w293:i32)
            n265 = Index Array(array=w308, index=w293) -> (element=w307:T19)
            n266 = local read "Specifiers On/Off"() -> (w298:T2)
            n267 = Unbundle By Name(w307) -> ("Specifier enabled"=w294:bool, "Condition type"=w290:T6, "Comparison type"=w306:T7, "Value"=w305:dbl, "Validity criteria(s)"=w304:T4)
            n268 = Cluster To Array(cluster=w298) -> (array=w297:bool[])
            n269 = Replace Array Subset(array=w297, new element=w294, index=w293) -> (w296:bool[])
            n270 = Index Array(array=w304, index=0) -> (element=w302:T20)
            n271 = local write "SubCondition type"(w290) -> ()
            n272 = local write "Comparison type"(w306) -> ()
            n273 = local write "Compare against"(w305) -> ()
            n274 = Array To Cluster(array=w296) -> (cluster=w295:T21)
            n275 = Unbundle By Name(w302) -> ("V. check enabled"=w300:bool, "Criteria"=w301:T3, "Validity value"=w299:dbl)
            n276 = local write "Specifiers On/Off"(w295) -> ()
            n277 = local write "Validity Enabled"(w300) -> ()
            n278 = local write "SC. Validity Criteria"(w301) -> ()
            n279 = local write "Valid for, units"(w299) -> ()
          }
          event "Discard and exit": Value Change {
            n280 = event-data() -> ("OldVal"=w311:bool)  [unwired: 1 in, 5 out]
            n281 = local write "Discard and exit"(w311) -> ()
            n282 = local read "Array of conditions in"() -> (w309:T12)
            n283 = local write "Array of conditions out"(w309) -> ()
          }
        }
      }
      "error out" <- w64
    }
    frame Enabled {
    }
  }
